vi "sub vi - Axis Channel.vi"(1 "Axis":u16(ring) items=["X", "Y", "Z"]) -> (0 "physical channels":tag="Dev1/ao0")   [LabVIEW 2010]
panel:
  # "About this Program:\n     - This sub-vi outputs the physical channel\n        corresponding to the axis"
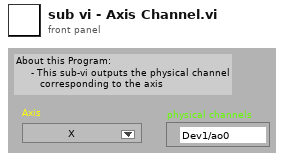
[diagram p1: front panel]
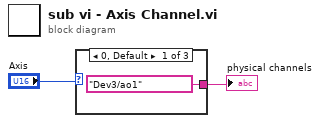
[diagram p0: block diagram]
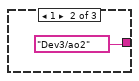
[diagram p2: hidden frame]
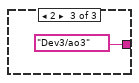
[diagram p3: hidden frame]
diagram:
  n1 = case shown="0, Default" "Axis" {
    tunnel: [tag "Dev3/ao1" ("physical channels") tag "Dev3/ao2" ("physical channels") tag "Dev3/ao3" ("physical channels")] -> w1
    frame 0, Default {
    }
    frame 1 {
    }
    frame 2 {
    }
  }
  "physical channels" <- w1
